vi "Move SmartMotor.vi"(0 "reference in":refnum<class "SmartMotor.lvclass">, 5 "error in (no error)":errorcluster) -> (14 "reference out":refnum<class "SmartMotor.lvclass">, 19 "error out":errorcluster)   [LabVIEW 2017, in "SmartMotor.lvclass"]
uses:
  SmartMotor.lvclass
  utils/SmartMotor Status.ctl
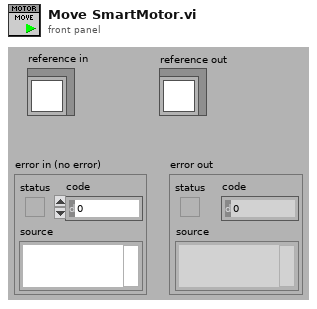
[diagram p1: front panel]
types:
  T1 = typedef "SmartMotor.lvclass/SmartMotor Status.ctl" = enum8{"Stopped", "Moving"}
  T2 = typedef "SmartMotor.lvclass/ObjectAttributes.ctl" = cluster{"SmartMotor Chain VISA Resource":refnum<visa-resource-name>, "SmartMotor Chain Address":i16, "Motor Absolute Position":i32, "Motor Relative Position":i32, "Motor Torque":i32, "Motor Voltage":i32, "Screwdriver Engaged":bool, "Screwdriver Torque Limit":i32, "Torque Monitor On/Off Status":bool, "Torque Monitor VI Reference":refnum<vi>, "Absolute Motor Torque (Filtered)":dbl, "SmartMotor Status":T1, "SmartMotor Error":T3}
  T3 = typedef "SmartMotor.lvclass/SmartMotor Error.ctl" = enum8{"None", "Read Error", "Low Voltage"}
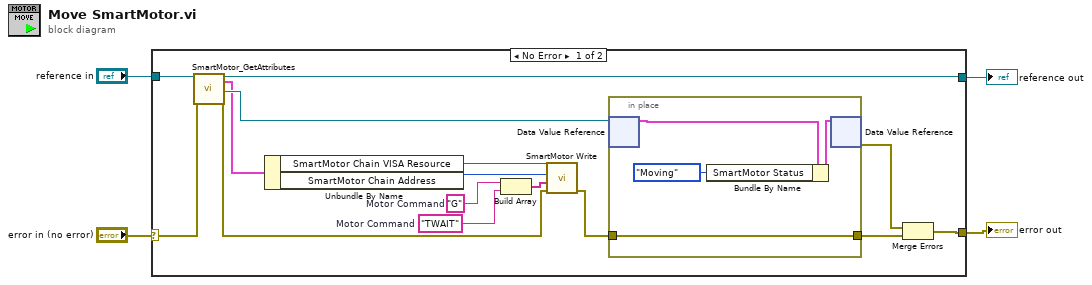
[diagram p0: block diagram]
diagram:
  n1 = case shown="No Error" "error in (no error)" {
    selector: "error in (no error)" -> [w18 w25]
    tunnel: [w15 w25] -> w3
    tunnel: [w16 w24] -> w1
    tunnel: "reference in" -> [w19 w24]
    frame No Error {
      w5 = "TWAIT"  # Motor Command
      w6 = "G"  # Motor Command
      n2 = call "SmartMotor_GetAttributes.vi"("reference in"=w19, "error in (no error)"=w18) -> ("reference out"=w16:refnum<class "SmartMotor.lvclass">, "Data"=w9:T2, "DataRef"=w14:refnum<data-value>, "error out"=w8:errorcluster)  [unwired: 14 in]
      n3 = Unbundle By Name(w9) -> ("SmartMotor Chain VISA Resource"=w11:refnum<visa-resource-name>, "SmartMotor Chain Address"=w10:i16)
      n4 = Build Array(w6, w5) -> (w12:string[])
      n5 = call "SmartMotor Write.vi"("VISA resource IN"=w11, "Motor Number"=w10, "Motor Command Array"=w12, "Error In"=w8) -> ("Error Out"=w7:errorcluster)  [unwired: 3 in, 2 out]
      n6 = in-place {
        in-place-border: w7 -> [w20]
        in-place-border: [w20] -> w13
        n7 = in-place-dvr #1(w14) -> (w22:T2)  [unwired: 1 out]
        n8 = Bundle By Name(cluster=w22, "SmartMotor Status"=SmartMotor_Status."Moving") -> (w23:T2)
        n9 = in-place-dvr #1(w23) -> (w17:errorcluster)  [unwired: 1 out]
      }
      n10 = Merge Errors(w17, w13) -> (w15:errorcluster)
    }
    frame Error {
    }
  }
  "error out" <- w3
  "reference out" <- w1
